vi "timing self-test.vi"() -> ()   [LabVIEW 2018]
uses:
  <vilib>/Platform/TimedLoop/XDataNode/timing_clust.ctl
  <vilib>/Platform/TimedLoop/XDataNode/nitl_modes.ctl
  <vilib>/Platform/TimedLoop/XDataNode/wakeup.ctl
  <vilib>/rvi/Emulation/niFpgaGetClockAttributes.vi
  <vilib>/rvi/Emulation/niFpgaSctlEmulationGetInTimedLoop.vi
  <vilib>/rvi/Emulation/niFpgaEmulationReportErrorSimple.vi
  <vilib>/rvi/Emulation/niFpgaProcessEmulError.vi
  <vilib>/rvi/Emulation/niFpgaCriticalErrorInLSC.vi
  <vilib>/rvi/eio/common/nirviEmuTemplateMethod_errors.vi
  <vilib>/rvi/interface/RandomDataEmulation/niFpgaRandomDataHandleErrors.vi
  <vilib>/platform/TimedLoop/XDataNode/XDataNode.xnode
  <vilib>/eio/EIONode/EIONode.xnode
  <vilib>/rvi/DataTransferAndStorage/Container/XNode/niFpgaContainer.xnode
  <vilib>/rvi/interface/RandomDataEmulation/nirviRandomDataFpgaReadWriteTemplate.vi
  <vilib>/Platform/TimedLoop/XDataNode/XDNodeRunTimeDep.lvlib
panel:
  in  "output freq (kHz)":sgl
  out "rising freq (kHz)":sgl
  out "falling freq (kHz)":sgl
  in  "STOP":bool
  out "rising period":u32
  out "falling period":u32
  in  "output cycles":u32
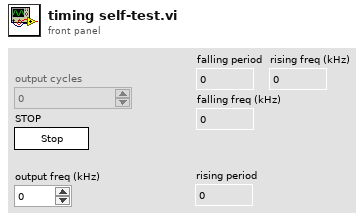
[diagram p1: front panel]
types:
  T1 = typedef "XDNodeRunTimeDep.lvlib/timing_clust.ctl" = cluster{"Expected End [f-1]":u64, "Actual End [f-1]":u64, "Finished Late? [f-1]":bool, "Expected End [i-1]":u64, "Actual End [i-1]":u64, "Finished Late? [i-1]":bool, "Expected Start [i]":u64, "Actual Start [i]":u64, "Expected Start [f]":u64, "Actual Start [f]":u64, "Source Name":string, "Structure Name":string, "Period":i64, "Deadline":i64, "Offset":i64, "Start":i64, "Priority":i32, "Timeout":i32, "Mode":T2, "Wakeup Reason":T3, "Error":errorcluster, "Source Type":string, "Secondary Source Type":string, "Global End Time":u64, "Global Start Time":u64, "Frame Duration":u64, "Iteration Duration":u64, "Assigned CPU":i32, "I/O Scan Engine Mode":u32}
  T2 = typedef "XDNodeRunTimeDep.lvlib/nitl_modes.ctl" = enum32{"No Change", "Process missed periods, maintain original phase", "Discard missed periods, maintain original phase", "Process missed periods, ignore original phase", "Discard missed periods, ignore original phase"}
  T3 = typedef "XDNodeRunTimeDep.lvlib/wakeup.ctl" = enum32{"Normal", "Aborted", "Asynchronous wakeup", "Timing source error", "Timed loop error", "Timeout"}
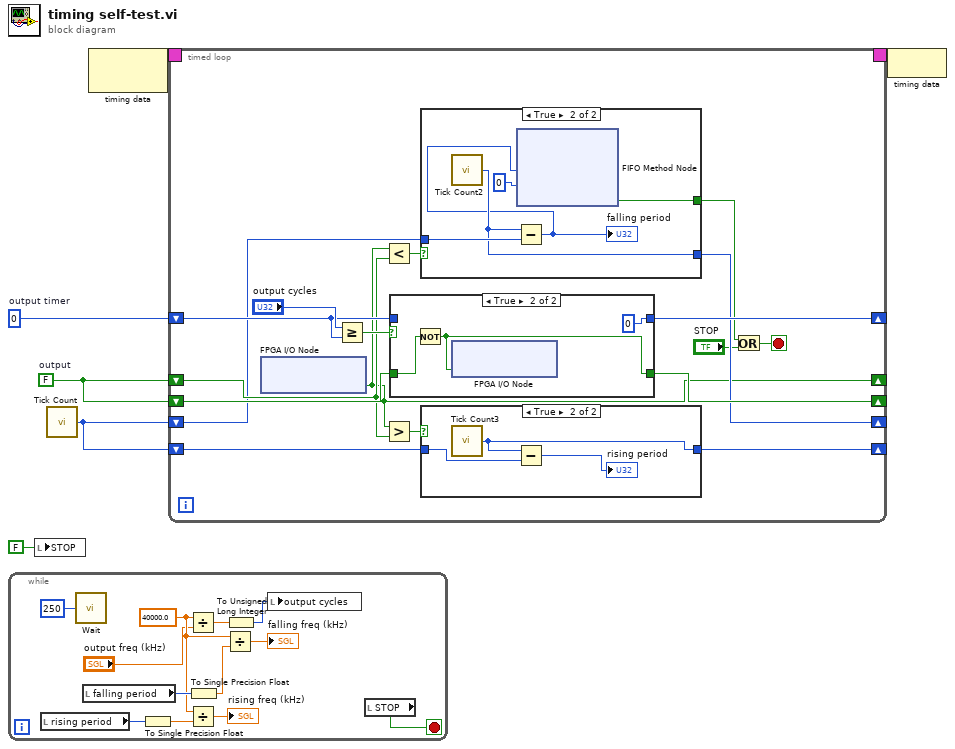
[diagram p0: block diagram]
diagram:
  w3 = FALSE  # output
  w4 = u32 0  # output timer
  n1 = while {
    stop <- w18 stop-if-true
    w10 = sgl 40000.0 ("y")
    n2 = local read "rising period"() -> (w15:u32)
    n3 = call "Wait"("Count(mSec)"=u16 250) -> ()  [unwired: 1 out]
    n4 = local read "falling period"() -> (w16:u32)
    n5 = To Single Precision Float(number=w15) -> (single precision float=w13:sgl)
    n6 = Divide(x=w10, y="output freq (kHz)") -> (x/y=w8:sgl)
    n7 = Divide(x=w10, y=w13) -> (x/y=→"rising freq (kHz)":sgl)
    n8 = To Single Precision Float(number=w16) -> (single precision float=w14:sgl)
    n9 = Divide(x=w10, y=w14) -> (x/y=→"falling freq (kHz)":sgl)
    n10 = To Unsigned Long Integer(number=w8) -> (unsigned 32bit integer=w7:u32)
    n11 = local write "output cycles"(w7) -> ()
    n12 = local read "STOP"() -> (w18:bool)
  }
  n13 = local write "STOP"(FALSE ("STOP")) -> ()
  n14 = call "Tick Count"() -> ("Tick Count(Ticks)"=w2:u32)
  n15 = node-c288() -> (w6:T1)  [unwired: 1 in]
  n16 = timed-loop {
    timing: w6 -> [_]
    timing-out: [_] -> w5
    shift-right: [w32] -> _
    shift-left: w4 -> [w33]
    shift-right: [w30] -> _
    shift-left: w3 -> [w31]
    shift-right: [w26] -> _
    shift-left: w2 -> [w27]
    shift-right: [w23] -> _
    shift-left: w2 -> [w24]
    shift-right: [w22] -> _
    shift-left: w3 -> [w29]
    stop <- w20 stop-if-true
    n17 = xnode "FPGA I/O Node"() -> ("Mod1/DIO0"=w22:bool)  [unwired: 1 in, 1 out]
    n18 = Greater Or Equal?(x="output cycles", y=w33) -> (x >= y?=w34:bool)
    n19 = Less?(x=w22, y=w29) -> (x < y?=w28:bool)
    n20 = Greater?(x=w22, y=w29) -> (0:w25:bool)
    n21 = case shown="True" w34 {
      tunnel: w33 -> [w47 _]
      tunnel: [w47 u32 0 ("output timer")] -> w32
      tunnel: w31 -> [w46 w49]
      tunnel: [w46 w48] -> w30
      frame False {
      }
      frame True {
        n22 = Not(x=w49) -> (.not. x?=w48:bool)
        n23 = xnode "FPGA I/O Node"("Mod1/DIO7"=w48) -> ()  [unwired: 1 in, 1 out]
      }
    }
    n24 = case shown="True" w28 {
      tunnel: w27 -> [w40 w45]
      tunnel: [w40 w44] -> w26
      tunnel: [_ w42] -> w19
      frame False {
      }
      frame True {
        n25 = call "Tick Count2"() -> ("Tick Count(Ticks)"=w44:u32)
        n26 = Subtract(x=w44, y=w45) -> (x-y=w41:u32)
        "falling period" <- w41
        n27 = xnode ("FIFO Method Node")("Element"=w41, "Timeout"=0) -> ("Timed Out?"=w42:bool)  [unwired: 1 in, 1 out]
      }
    }
    n28 = case shown="True" w25 {
      tunnel: w24 -> [w36 w39]
      tunnel: [w36 w37] -> w23
      frame False {
      }
      frame True {
        n29 = call "Tick Count3"() -> ("Tick Count(Ticks)"=w37:u32)
        n30 = Subtract(x=w37, y=w39) -> (x-y=→"rising period":u32)
      }
    }
    n31 = Or(x=w19, y="STOP") -> (x .or. y?=w20:bool)
  }
  n32 = node-c288(w5) -> ()
